vi "FPGA_sine.vi"(0 "Update Freq (Hz)":dbl, 1 "Phase (Deg)":dbl, 2 "Frequency (Hz)":dbl, 3 "Amplitude (V)":dbl) -> ()   [LabVIEW 2009]
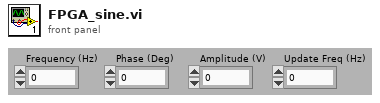
[diagram p1: front panel]
types:
  T1 = enum32{"Invalid", "Standard", "Closed", "Hidden", "Minimized", "Maximized"}
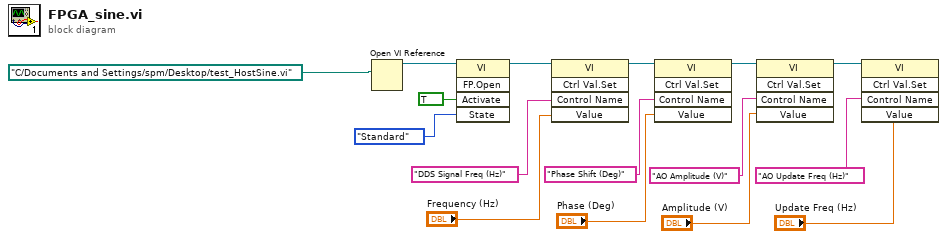
[diagram p0: block diagram]
diagram:
  n1 = Open VI Reference(vi path=path "C:/Documents and Settings/spm/Desktop/test_HostSine.vi") -> (vi reference=w16:refnum<vi>)  [unwired: 5 in, 1 out]
  n2 = invoke class="VI" method="FP.Open"(reference=w16, "Activate"=TRUE, "State"=T1."Standard") -> (reference out=w12:refnum<vi>)  [unwired: 2 in, 4 out]
  n3 = invoke class="VI" method="Ctrl Val.Set"(reference=w12, "Control Name"="DDS Signal Freq (Hz)", "Value"="Frequency (Hz)") -> (reference out=w11:refnum<vi>)  [unwired: 2 in, 4 out]
  n4 = invoke class="VI" method="Ctrl Val.Set"(reference=w11, "Control Name"="Phase Shift (Deg)", "Value"="Phase (Deg)") -> (reference out=w10:refnum<vi>)  [unwired: 2 in, 4 out]
  n5 = invoke class="VI" method="Ctrl Val.Set"(reference=w10, "Control Name"="AO Amplitude (V)", "Value"="Amplitude (V)") -> (reference out=w9:refnum<vi>)  [unwired: 2 in, 4 out]
  n6 = invoke class="VI" method="Ctrl Val.Set"(reference=w9, "Control Name"="AO Update Freq (Hz)", "Value"="Update Freq (Hz)") -> ()  [unwired: 2 in, 5 out]
